vi "Saturation_Counter.vi"(10 "Filtered Output":dbl, 11 "Saturation Limit":sgl) -> ()   [LabVIEW 2014]
uses:
  Saturation_Count.vi
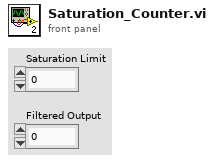
[diagram p1: front panel]
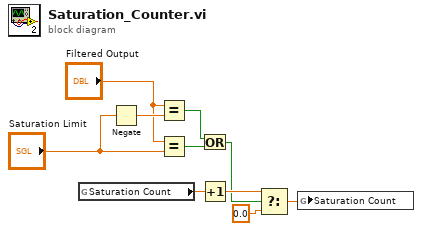
[diagram p0: block diagram]
diagram:
  n1 = global read "Saturation_Count.vi" "Saturation Count"() -> (w8:dbl)
  n2 = Negate(x="Saturation Limit") -> (-x=w9:sgl)
  n3 = Equal?(x="Filtered Output", y=w9) -> (x = y?=w3:bool)
  n4 = Equal?(x="Filtered Output", y="Saturation Limit") -> (x = y?=w4:bool)
  n5 = Or(x=w3, y=w4) -> (x .or. y?=w1:bool)
  n6 = Increment(x=w8) -> (x+1=w5:dbl)
  n7 = Select(t=w5, s=w1, f=0.0) -> (s? t:f=w7:dbl)
  n8 = global write "Saturation_Count.vi" "Saturation Count"(w7) -> ()
